vi "VLD_clustering_xy_sub.vi"(10 "x,y 배열":cluster{"x":dbl, "y":dbl}[](array[cluster])) -> (0 "steer":dbl, 1 "전체 관찰용":cluster{cluster{"x":dbl, "y":dbl}[]}[](array[cluster]), 2 "xy 1d clust":cluster{"x":dbl, "y":dbl}[](array[cluster]), 3 "주행 관찰용":cluster{cluster{"x":dbl, "y":dbl}[]}[](array[cluster]))   [LabVIEW 2015]
panel:
  out "XY 그래프 5":cluster{cluster{"x":dbl, "y":dbl}[]}[](graph)
  out "XY 그래프 3":cluster{"x":dbl, "y":dbl}[](graph)
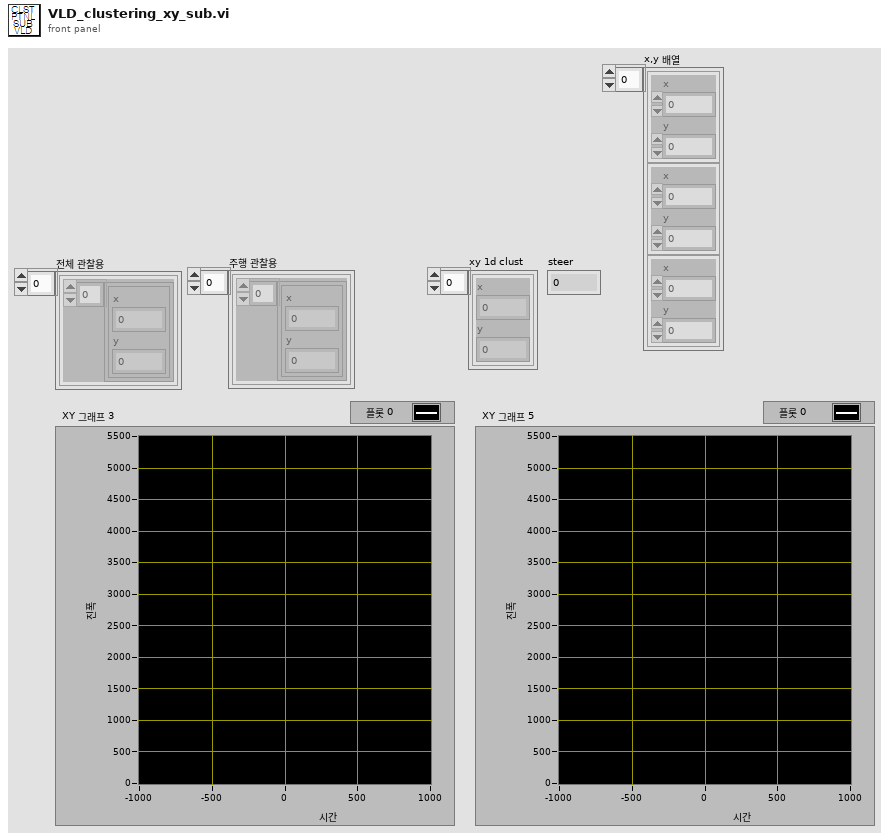
[diagram p1: front panel]
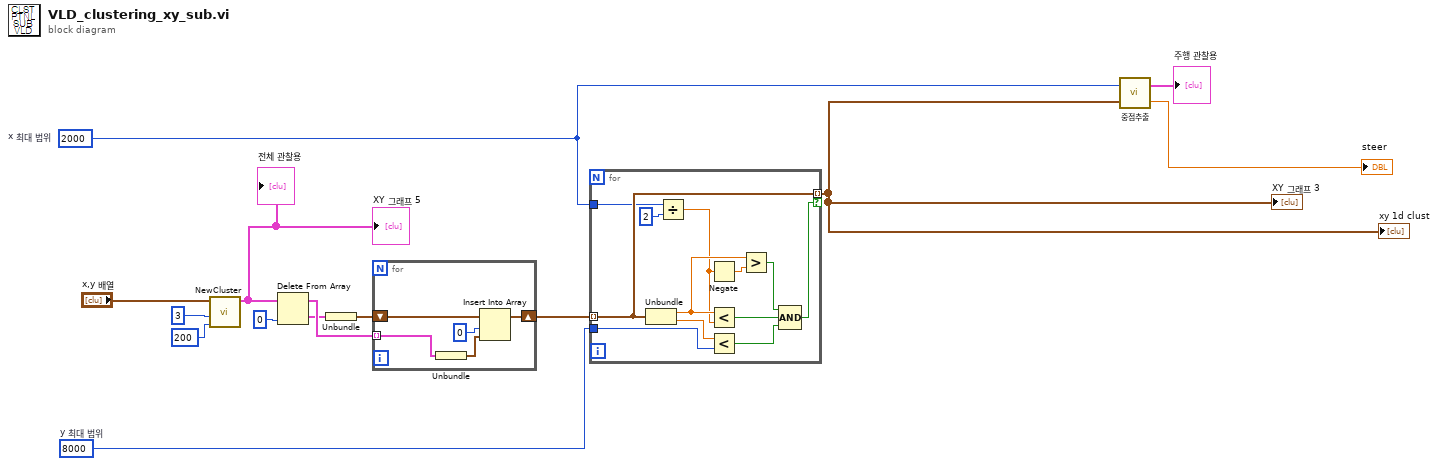
[diagram p0: block diagram]
diagram:
  w7 = 2000  # x 최대 범위
  w9 = 8000  # y 최대 범위
  n1 = call "NewCluster.vi"("R_th"=200, "군집 원소 최수 개수"=3, "x,y 배열"="x,y 배열") -> ("클러스터링된 점 배열"=w2:cluster{cluster{"x":dbl, "y":dbl}[]}[])  [unwired: 8 in]
  "XY 그래프 5" <- w2
  "전체 관찰용" <- w2
  n2 = Delete From Array(array=w2, index=0 ("인덱스")) -> (deleted portion=w11:cluster{cluster{"x":dbl, "y":dbl}[]}, array with subset deleted=w14:cluster{cluster{"x":dbl, "y":dbl}[]}[])  [unwired: 1 in]
  n3 = Unbundle(w11) -> (w12:cluster{"x":dbl, "y":dbl}[])
  n4 = for {
    tunnel: w14 -> [w19] mode=indexing
    shift-right: [w16] -> w10
    shift-left: w12 -> [w15]
    n5 = Unbundle(w19) -> (w18:cluster{"x":dbl, "y":dbl}[])
    n6 = Insert Into Array(array=w15, index=0 ("인덱스"), new element=w18) -> (w16:cluster{"x":dbl, "y":dbl}[])
  }
  n7 = for {
    tunnel: w10 -> [w29] mode=indexing
    tunnel: w7 -> [w28]
    tunnel: w9 -> [w30]
    tunnel: [w29] -> w8 mode=indexing if=w20
    n8 = Unbundle(w29) -> ("x"=w26:dbl, "y"=w31:dbl)
    n9 = Divide(x=w28, y=2) -> (x/y=w24:dbl)
    n10 = Negate(x=w24) -> (-x=w25:dbl)
    n11 = Less?(x=w26, y=w24) -> (x < y?=w22:bool)
    n12 = Less?(x=w31, y=w30) -> (x < y?=w23:bool)
    n13 = Greater?(x=w26, y=w25) -> (0:w21:bool)
    n14 = Compound Arithmetic op=AND ("복합 연산")(w21, w22, w23) -> (w20:bool)
  }
  "XY 그래프 3" <- w8
  "xy 1d clust" <- w8
  n15 = call "중점추출.vi"("x,y 배열"=w8, "x범위"=w7) -> ("steer"=→"steer":dbl, "주행 관찰용"=→"주행 관찰용":cluster{cluster{"x":dbl, "y":dbl}[]}[])
